vi "Focus Tip.vi"(0 "Focus Tip":refnum<vi>, 1 "Image Analysis":T1, 2 "Indicators":T2, 5 "Focusing Parameters":T3, 9 "Image Area":cluster{"Width":i32, "Height":i32}, 11 "error in (no error)":errorcluster, 12 "Transformation Matrix":refnum<vi>, 13 "Indicator":refnum<vi>, 14 "Abort":refnum<vi>) -> (15 "error out":errorcluster)   [LabVIEW 2012, in "Visual Analyser.lvlib"]
uses:
  Visual Analyser.lvlib
  <vilib>/Analysis/Matrix/Datatypes/RealMatrix.ctl
  <vilib>/Analysis/Matrix/NI_Matrix.lvlib
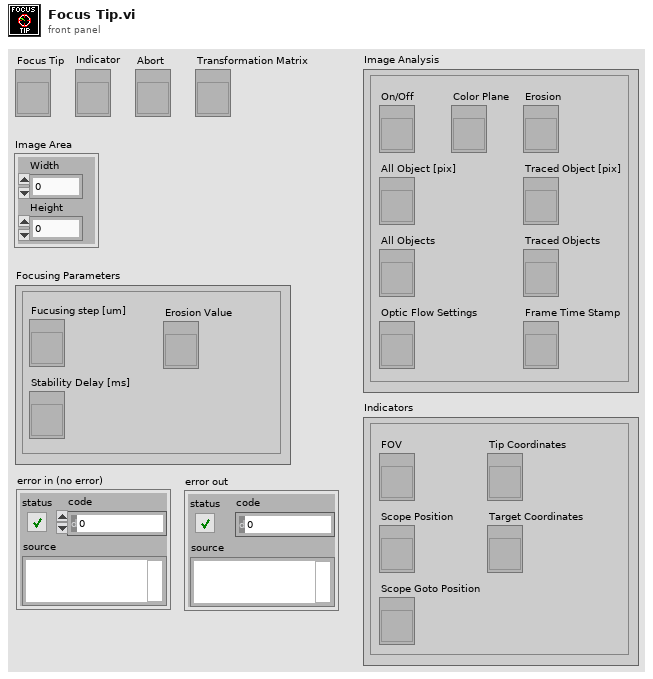
[diagram p1: front panel]
types:
  T1 = cluster{"On/Off":refnum<vi>, "All Objects":refnum<vi>, "Color Plane":refnum<vi>, "Erosion":refnum<vi>, "Traced Objects":refnum<vi>, "Frame Time Stamp":refnum<vi>, "Optic Flow Settings":refnum<vi>, "All Object [pix]":refnum<vi>, "Traced Object [pix]":refnum<vi>}
  T2 = cluster{"Tip Coordinates":refnum<vi>, "Target Coordinates":refnum<vi>, "Scope Position":refnum<vi>, "FOV":refnum<vi>, "Scope Goto Position":refnum<vi>}
  T3 = cluster{"Erosion Value":refnum<vi>, "Fucusing step [um]":refnum<vi>, "Stability Delay [ms]":refnum<vi>}
  T4 = cluster{"Area":dbl, "Centre of Mass":cluster{"X":dbl, "Y":dbl}, "Global Rectangle":cluster{"Left":dbl, "Top":dbl, "Right":dbl, "Bottom":dbl}, "Contrast":dbl}[]
  T5 = cluster{"Area":dbl, "Centre of Mass":cluster{"X":dbl, "Y":dbl}, "Global Rectangle":cluster{"Left":dbl, "Top":dbl, "Right":dbl, "Bottom":dbl}, "Contrast":dbl}
  T6 = cluster{"X [um]":dbl, "Y [um]":dbl, "Z [um]":dbl}
  T7 = cluster{"X [um]":bool, "Y [um]":bool, "Z [um]":bool}
  T8 = typedef "NI_Matrix.lvlib/RealMatrix.ctl" = dbl[][]
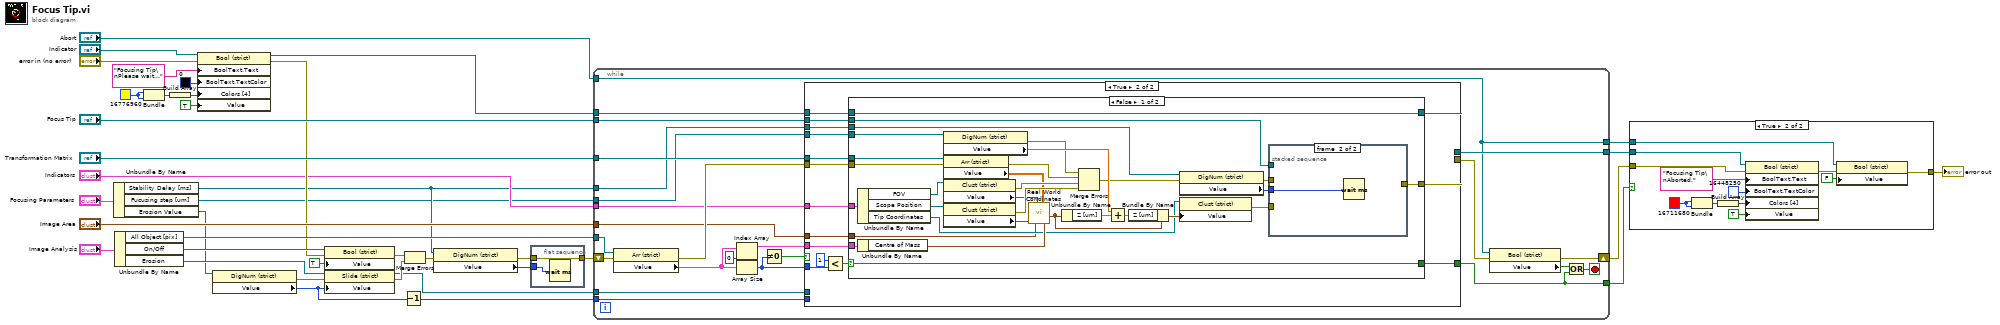
[diagram p0: block diagram]
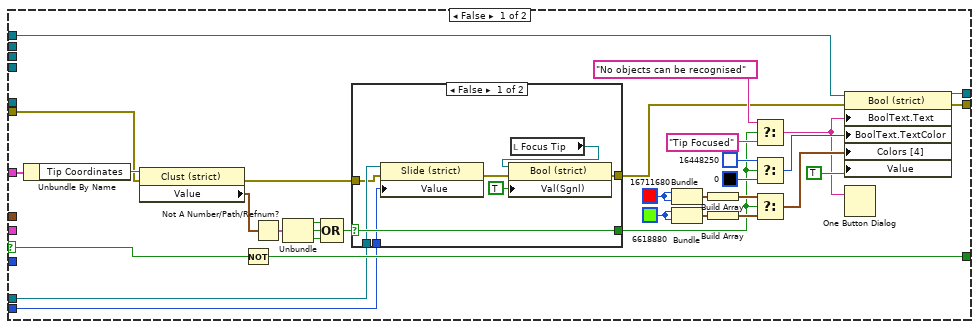
[diagram p3: hidden frame]
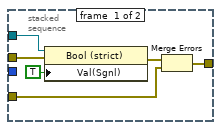
[diagram p5: hidden frame]
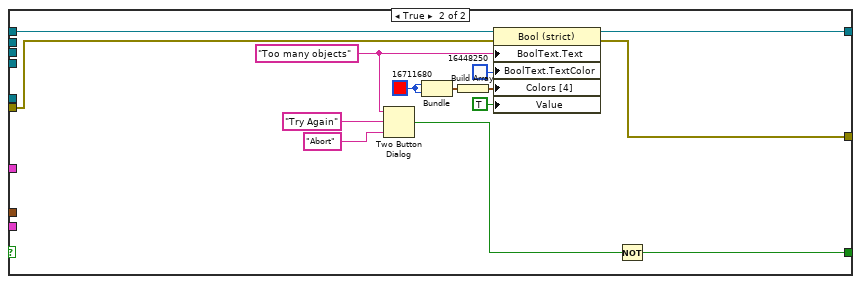
[diagram p6: hidden frame]
diagram:
  w35 = u32 16776960
  n1 = Unbundle By Name("Focusing Parameters") -> ("Stability Delay [ms]"=w3:refnum<vi>, "Fucusing step [um]"=w2:refnum<vi>, "Erosion Value"=w9:refnum<vi>)
  n2 = Unbundle By Name("Image Analysis") -> ("All Object [pix]"=w27:refnum<vi>, "On/Off"=w26:refnum<vi>, "Erosion"=w24:refnum<vi>)
  n3 = Bundle(w35, w35) -> (w36:cluster{u32, u32})  [unwired: 1 in]
  n4 = Build Array(w36) -> (w34:cluster{u32, u32}[])
  n5 = property class="Bool (strict)"(reference="Indicator", error in="error in (no error)", "BoolText.Text"="Focusing Tip\nPlease wait..." ("Window Title (\"\")"), "BoolText.TextColor"=u32 0, "Colors [4]"=w34, "Value"=TRUE ("Visible")) -> (reference out=w30:refnum<vi>, error out=w7:errorcluster)
  n6 = property on="Property Node" class="DigNum (strict)"(reference=w9) -> (error out=w21:errorcluster, "Value"=w17:u32)  [unwired: 1 in, 1 out]
  n7 = property on="Property Node" class="Bool (strict)"(reference=w26, error in=w7, "Value"=TRUE) -> (error out=w25:errorcluster)  [unwired: 1 out]
  n8 = property on="Property Node" class="Slide (strict)"(reference=w24, error in=w21, "Value"=w17) -> (reference out=w14:refnum<vi>, error out=w23:errorcluster)
  n9 = Decrement(x=w17) -> (x-1=w16:u32)
  n10 = Merge Errors(w25, w23) -> (w20:errorcluster)
  n11 = property on="Property Node" class="DigNum (strict)"(reference=w3, error in=w20) -> (error out=w19:errorcluster, "Value"=w18:u32)  [unwired: 1 out]
  n12 = flat-sequence {
    tunnel: [w41] -> w8
    tunnel: w19 -> [w41]
    tunnel: w18 -> [w40]
    frame #0 {
      n13 = Wait (ms)(milliseconds to wait=w40) -> ()  [unwired: 1 out]
    }
  }
  n14 = while {
    tunnel: w27 -> [w65]
    tunnel: w30 -> [w62]
    shift-right: [w46] -> w29
    shift-left: w8 -> [w47]
    tunnel: [w59] -> w28
    tunnel: w14 -> [w56]
    tunnel: w16 -> [w55]
    tunnel: "Indicators" -> [w53]
    tunnel: "Transformation Matrix" -> [w52]
    tunnel: w2 -> [w51]
    tunnel: w3 -> [w50]
    tunnel: [w43] -> w13
    tunnel: "Focus Tip" -> [w49]
    tunnel: "Image Area" -> [w48]
    tunnel: "Abort" -> [w42]
    tunnel: [w42] -> w5
    stop <- w60 stop-if-true
    n15 = property on="Property Node" class="Arr (strict)"(reference=w65, error in=w47) -> (error out=w61:errorcluster, "Value"=w54:T4)  [unwired: 1 out]
    n16 = Index Array(array=w54, index=0 ("disabled index (col)")) -> (element=w63:T5)
    n17 = Array Size(array=w54) -> (size(s)=w64:i32)
    n18 = Not Equal To 0?(x=w64) -> (x != 0?=w57:bool)
    n19 = case shown="True" w57 {
      selector: w57 -> [w76 _]
      tunnel: w64 -> [_ w111]
      tunnel: w63 -> [_ w123]
      tunnel: w62 -> [w81 w122]
      tunnel: [w67 w109] -> w45
      tunnel: w61 -> [w66 w117]
      tunnel: [w75 w121] -> w43
      tunnel: [w74 w120] -> w59
      tunnel: w56 -> [w73 _]
      tunnel: w55 -> [w72 _]
      tunnel: w53 -> [w71 w118]
      tunnel: w52 -> [_ w116]
      tunnel: w51 -> [_ w115]
      tunnel: w50 -> [_ w114]
      tunnel: w49 -> [_ w113]
      tunnel: w48 -> [_ w112]
      frame False {
        w85 = u32 6618880
        w98 = u32 16711680
        n20 = Unbundle By Name(w71) -> ("Tip Coordinates"=w70:refnum<vi>)
        n21 = property on="Property Node" class="Clust (strict)"(reference=w70, error in=w66) -> (error out=w69:errorcluster, "Value"=w78:T6)  [unwired: 1 out]
        n22 = Not(x=w76) -> (.not. x?=w75:bool)
        n23 = Not A Number/Path/Refnum?(number/path/refnum=w78) -> (NaN/Path/Refnum?=w92:T7)
        n24 = Unbundle(w92) -> ("X [um]"=w93:bool, "Y [um]"=w94:bool, "Z [um]"=w95:bool)
        n25 = Compound Arithmetic op=OR(w93, w94, w95) -> (w79:bool)
        n26 = case shown="False" w79 {
          selector: w79 -> [w106 w108]
          tunnel: [w106 w108] -> w77
          tunnel: [w104 w107] -> w68
          tunnel: w73 -> [w101 _]
          tunnel: w72 -> [w100 _]
          tunnel: w69 -> [w99 w107]
          frame False {
            n27 = property on="Property Node" class="Slide (strict)"(reference=w101, error in=w99, "Value"=w100) -> (error out=w102:errorcluster)  [unwired: 1 out]
            n28 = local read "Focus Tip"() -> (w103:refnum<vi>)
            n29 = property on="Property Node" class="Bool (strict)"(reference=w103, error in=w102, "Val(Sgnl)"=TRUE ("Value (Signaling)")) -> (error out=w104:errorcluster)  [unwired: 1 out]
          }
          frame True {
          }
        }
        n30 = Bundle(w98, w98) -> (w97:cluster{u32, u32})  [unwired: 1 in]
        n31 = Bundle(w85, w85) -> (w86:cluster{u32, u32})  [unwired: 1 in]
        n32 = Build Array(w97) -> (w84:cluster{u32, u32}[])
        n33 = Build Array(w86) -> (w83:cluster{u32, u32}[])
        n34 = Select(t="No objects can be recognised" ("message"), s=w77, f="Tip Focused" ("message")) -> (s? t:f=w80:string)
        n35 = Select(t=u32 16448250, s=w77, f=u32 0) -> (s? t:f=w87:u32)
        n36 = Select(t=w84, s=w77, f=w83) -> (s? t:f=w82:cluster{u32, u32}[])
        n37 = property class="Bool (strict)"(reference=w81, error in=w68, "BoolText.Text"=w80, "BoolText.TextColor"=w87, "Colors [4]"=w82, "Value"=TRUE ("Visible")) -> (reference out=w74:refnum<vi>, error out=w67:errorcluster)
        n38 = One Button Dialog(message=w80) -> ()  [unwired: 1 in, 1 out]
      }
      frame True {
        n39 = Less?(x=1 ("y"), y=w111) -> (x < y?=w119:bool)
        n40 = case shown="False" w119 {
          selector: w119 -> [w154 _]
          tunnel: w123 -> [w152 _]
          tunnel: w122 -> [w153 w170]
          tunnel: [w137 w166] -> w109
          tunnel: [w154 w164] -> w121
          tunnel: [w153 w163] -> w120
          tunnel: w118 -> [w150 _]
          tunnel: w117 -> [w127 w162]
          tunnel: w116 -> [w140 _]
          tunnel: w115 -> [w136 _]
          tunnel: w114 -> [w139 _]
          tunnel: w113 -> [w135 _]
          tunnel: w112 -> [w126 _]
          frame False {
            n41 = Unbundle By Name(w150) -> ("FOV"=w141:refnum<vi>, "Scope Position"=w143:refnum<vi>, "Tip Coordinates"=w142:refnum<vi>)
            n42 = Unbundle By Name(w152) -> ("Centre of Mass"=w151:cluster{"X":dbl, "Y":dbl})
            n43 = property on="Property Node" class="DigNum (strict)"(reference=w136) -> (error out=w128:errorcluster, "Value"=w144:dbl)  [unwired: 1 in, 1 out]
            n44 = property on="Property Node" class="Arr (strict)"(reference=w140, error in=w127) -> (error out=w132:errorcluster, "Value"=w130:T8)  [unwired: 1 out]
            n45 = property on="Property Node" class="Clust (strict)"(reference=w141) -> (error out=w133:errorcluster, "Value"=w131:cluster{"FOVx [um]":dbl, "FOVy [um]":dbl})  [unwired: 1 in, 1 out]
            n46 = property on="Property Node" class="Clust (strict)"(reference=w143) -> (error out=w134:errorcluster, "Value"=w149:T6)  [unwired: 1 in, 1 out]
            n47 = call "Real World Corrdinates.vi"("Transformation Matrix"=w130, "coordinates [pix]"=w151, "FOV"=w131, "Scope Position"=w149, "Image Area"=w126) -> ("Target Coordinates"=w147:T6)  [unwired: 6 in]
            n48 = Unbundle By Name(w147) -> ("Z [um]"=w146:dbl)
            n49 = Merge Errors(w128, w132, w133, w134) -> (w129:errorcluster)
            n50 = Add(x=w144, y=w146) -> (x+y=w145:dbl)
            n51 = Bundle By Name(cluster=w147, "Z [um]"=w145) -> (w148:T6)
            n52 = property on="Property Node" class="DigNum (strict)"(reference=w139, error in=w129) -> (error out=w125:errorcluster, "Value"=w138:u32)  [unwired: 1 out]
            n53 = property on="Property Node" class="Clust (strict)"(reference=w142, "Value"=w148) -> (error out=w124:errorcluster)  [unwired: 1 in, 1 out]
            n54 = stacked-sequence {
              tunnel: w138 -> [_ w161]
              tunnel: [w155 _] -> w137
              tunnel: w135 -> [w159 _]
              tunnel: w125 -> [w158 _]
              tunnel: w124 -> [w156 _]
              frame #0 {
                n55 = property on="Property Node" class="Bool (strict)"(reference=w159, error in=w158, "Val(Sgnl)"=TRUE ("Value (Signaling)")) -> (error out=w157:errorcluster)  [unwired: 1 out]
                n56 = Merge Errors(w157, w156) -> (w155:errorcluster)
              }
              frame #1 {
                n57 = Wait (ms)(milliseconds to wait=w161) -> ()  [unwired: 1 out]
              }
            }
          }
          frame True {
            w172 = u32 16711680
            w167 = "Too many objects" ("Window Title (\"\")")
            n58 = Two Button Dialog(message=w167, 1:"Abort" ("F button name (\"Cancel\")"), 2:"Try Again" ("T button name (\"OK\")")) -> (T button?=w165:bool)
            n59 = Bundle(w172, w172) -> (w173:cluster{u32, u32})  [unwired: 1 in]
            n60 = Build Array(w173) -> (w171:cluster{u32, u32}[])
            n61 = property class="Bool (strict)"(reference=w170, error in=w162, "BoolText.Text"=w167, "BoolText.TextColor"=u32 16448250, "Colors [4]"=w171, "Value"=TRUE ("Visible")) -> (reference out=w163:refnum<vi>, error out=w166:errorcluster)
            n62 = Not(x=w165) -> (.not. x?=w164:bool)
          }
        }
      }
    }
    n63 = property on="Property Node" class="Bool (strict)"(reference=w42, error in=w45) -> (error out=w46:errorcluster, "Value"=w44:bool)  [unwired: 1 out]
    n64 = Or(x=w44, y=w43) -> (x .or. y?=w60:bool)
  }
  n65 = case shown="True" w13 {
    tunnel: w29 -> [w176 w181]
    tunnel: w28 -> [_ w180]
    tunnel: [w176 w178] -> w31
    tunnel: w5 -> [_ w177]
    frame False {
    }
    frame True {
      w183 = u32 16711680
      n66 = Bundle(w183, w183) -> (w184:cluster{u32, u32})  [unwired: 1 in]
      n67 = Build Array(w184) -> (w182:cluster{u32, u32}[])
      n68 = property class="Bool (strict)"(reference=w180, error in=w181, "BoolText.Text"="Focusing Tip\nAborted." ("Window Title (\"\")"), "BoolText.TextColor"=u32 16448250, "Colors [4]"=w182, "Value"=TRUE ("Visible")) -> (error out=w179:errorcluster)  [unwired: 1 out]
      n69 = property on="Property Node" class="Bool (strict)"(reference=w177, error in=w179, "Value"=FALSE) -> (error out=w178:errorcluster)  [unwired: 1 out]
    }
  }
  "error out" <- w31
